vi "DMM_control.vi"(0 "Data in":string, 3 "error in":errorcluster) -> (5 "Data out":string="0.000764", 6 "millisecond timer value":u32, 8 "error out":errorcluster)   [LabVIEW 2011]
doc: "Data in:\n<function><nodes><resolution><range><autozero>\n\nFunction [Integer]\n 0 = DC Volts\n 1 = AC Volts\n 2 = DC Current\n 3 = AC Current\n 4 = Resistance (2 wire)\n 5 = Resistance (4 wire)\n 6 = Frequency\n 7 = Period\n 8 = Diode\n\nNodes [String]\n AB = measueres between a and b\n\nResolution [Integer]\n 0 = 3.5\n 1 = 4.5\n 2 = 5.5\n 3 = 6.5\n\nRange [Float]\n -1 = Autorange\n\nAutoZero [Integer]\n -1 = Auto\n 0 = Off (Default)\n 1 = On\n 2 = Once"
uses:
  <instrlib>/niDMM/nidmm.llb/niDMM Function.ctl
  Server_Globals.vi
  <instrlib>/niDMM/nidmm.llb/niDMM Configure Measurement Digits.vi
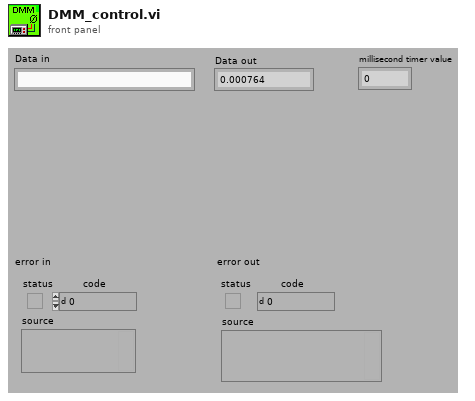
[diagram p1: front panel]
types:
  T1 = cluster{"I/O Settings":u64[], "Instrument Handle":cluster{"5402":refnum<k15>, " 5112":refnum<k15>, "4072":refnum<k15>, "USB":refnum<visa-resource-name>, "4110":refnum<k15>}, "Logfile":refnum<file>, "Log Level":i8, "Clear":i32[], "OS Set":cluster{"instrument handle out":refnum<k15>, "remaining string":string, "Settings":cluster{"Horizontal Conf.":cluster{"Min. Sample rate":dbl, "Reference position":dbl, "Record Length":i16}, "Channel A":cluster{"Enable":bool, "Vertical coupling":dbl, "Vertical range":dbl, "Vertical offset":dbl, "Probe attenuation":dbl}, "Channel B":cluster{"Enable":bool, "Vertical coupling":dbl, "Vertical range":dbl, "Vertical offset":dbl, "Probe attenuation":dbl}, "Trigger":cluster{"Source":enum8{"channel 1", "channel 2", "Imediate", "External trigger"}, "Slope":enum8{"Positive", "Negative"}, "Coupling":enum8{"AC", "DC"}, "Level":dbl, "Holdoff":dbl, "Delay":dbl, " Timeout":dbl, " Mode":enum8{"Normal", "Auto", "Auto Level"}}, "Measurements":cluster{"Measurement 1, Channel":enum8{"Channel 1", "Channel 2", "Channel 3", "Channel 4"}, "Measurement 1, Selection":u16, "Measurement 2, Channel":enum8{"Channel 1", "Channel 2", "Channel 3", "Channel 4"}, "Measurement 2,  Selection":u16, "Measurement 3, Channel":enum8{"Channel 1", "Channel 2", "Channel 3", "Channel 4"}, "Measurement 3, Selection 3":u16}}}, "DC Power Supply":cluster{"0":refnum<k15>, "1":refnum<k15>, "2":refnum<k15>, "3":refnum<k15>, "4":refnum<k15>}, "USB Interface":cluster{"0":refnum<visa-resource-name>, "1":refnum<visa-resource-name>, "2":refnum<visa-resource-name>, "3":refnum<visa-resource-name>, "4":refnum<visa-resource-name>}, "Function Generator":cluster{"0":refnum<k15>, "1":refnum<k15>, "2":refnum<k15>, "3":refnum<k15>, "4":refnum<k15>}, "Digital Multimeter":cluster{"0":refnum<k15>, "1":refnum<k15>, "2":refnum<k15>, "3":refnum<k15>, "4":refnum<k15>}, "Digital Osciliscope":cluster{"0":refnum<k15>, "1":refnum<k15>, "2":refnum<k15>, "3":refnum<k15>, "4":refnum<k15>}, "To M Server":string, "Adres":string[][], "Matrix version":string, "MD5":string, "Digital Multimeter Card 2":cluster{"0":string, "1":string, "2":string, "3":string, "4":string}}
  T2 = cluster{"0":refnum<k15>, "1":refnum<k15>, "2":refnum<k15>, "3":refnum<k15>, "4":refnum<k15>}
  T3 = typedef "niDMM Function.ctl" = enum16{"DC Volts", "AC Volts", "DC Current", "AC Current", "2-wire Resistance", "4-wire Resistance", "Diode", "Frequency", "Period", "AC Volts DC Coupled", "Capacitance", "Inductance", "Temperature"}
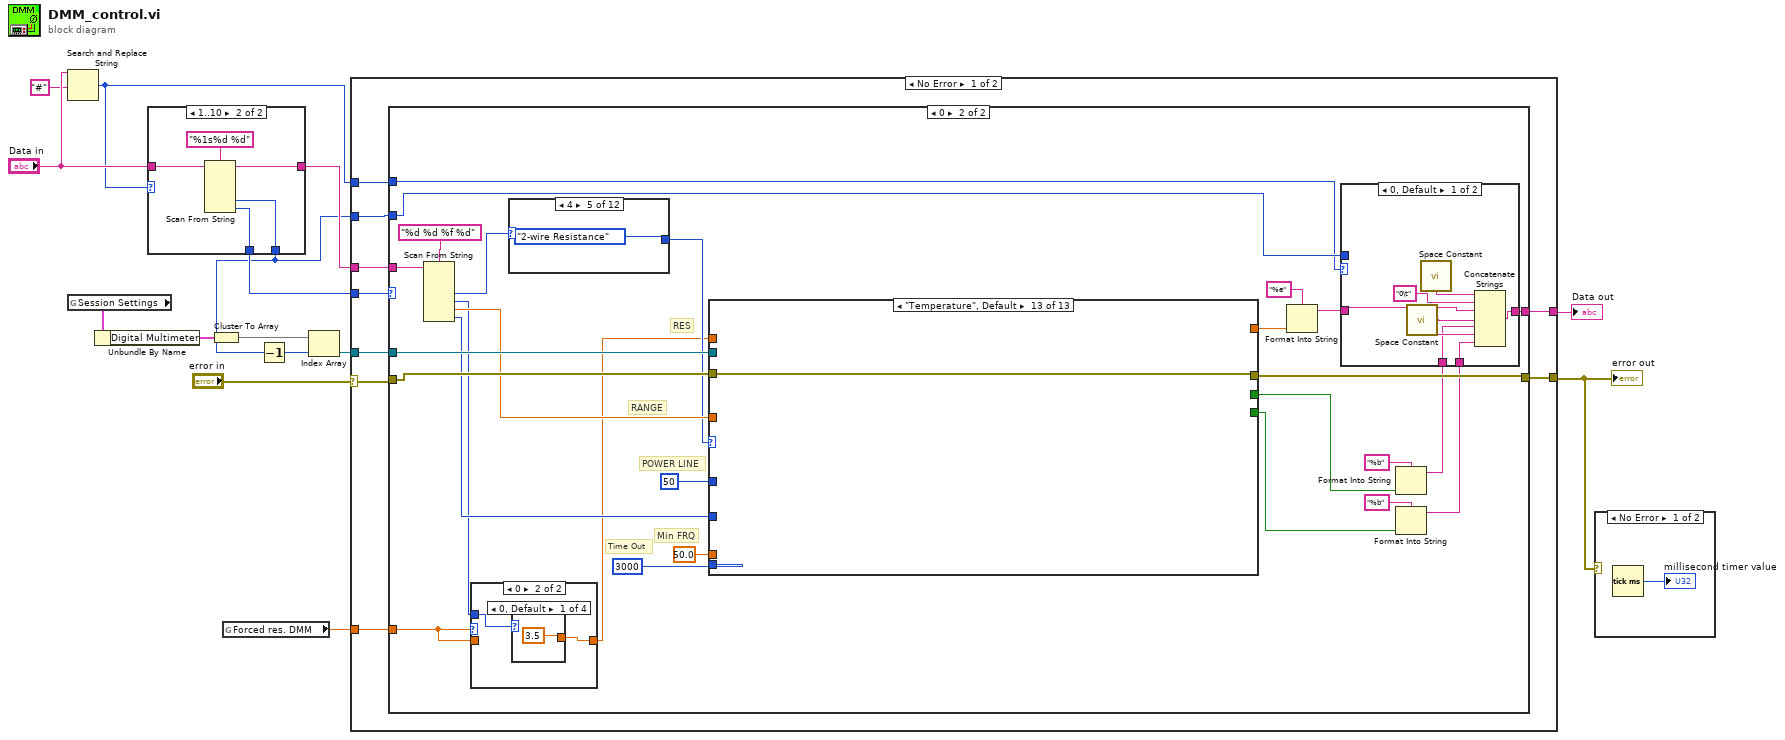
[diagram p0: block diagram]
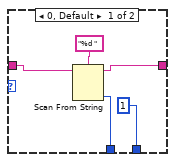
[diagram p2: hidden frame]
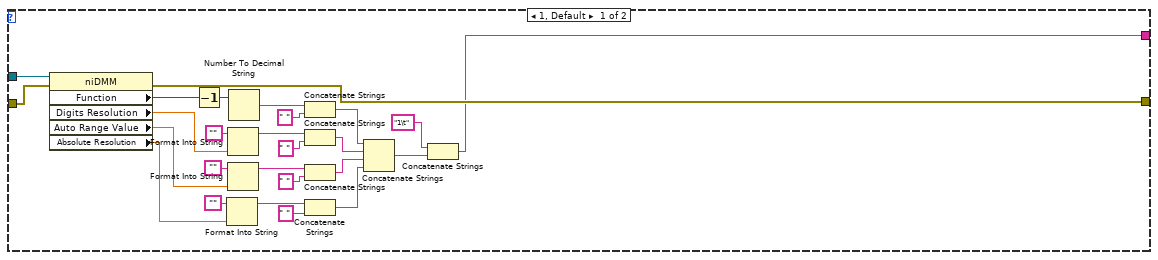
[diagram p4: hidden frame]
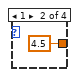
[diagram p6: hidden frame]
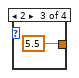
[diagram p7: hidden frame]
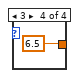
[diagram p8: hidden frame]
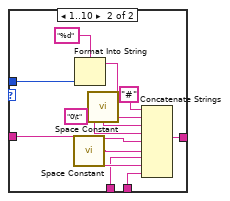
[diagram p9: hidden frame]
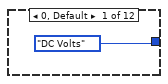
[diagram p10: hidden frame]
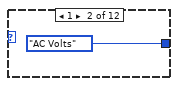
[diagram p11: hidden frame]
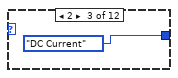
[diagram p12: hidden frame]
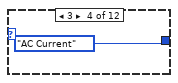
[diagram p13: hidden frame]
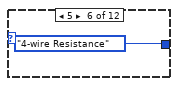
[diagram p14: hidden frame]
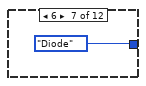
[diagram p15: hidden frame]
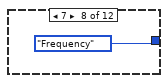
[diagram p16: hidden frame]
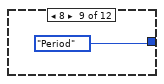
[diagram p17: hidden frame]
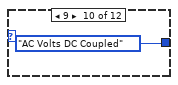
[diagram p18: hidden frame]
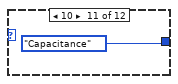
[diagram p19: hidden frame]
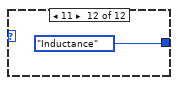
[diagram p20: hidden frame]
diagram:
  w3 = "#"
  n1 = Search and Replace String(input string="Data in", search string=w3, replace string=w3) -> (number of replacements=w2:i32)  [unwired: 5 in, 3 out]
  n2 = global read "Server_Globals.vi" "Session Settings"() -> (w12:T1)
  n3 = Unbundle By Name(w12) -> ("Digital Multimeter"=w11:T2)
  n4 = case shown="1..10" w2 {
    tunnel: [w19 w24] -> w15
    tunnel: [w16 w23] -> w7
    tunnel: [1 w22] -> w5
    tunnel: "Data in" -> [w20 w21]
    frame 0, Default {
      n5 = Scan From String(format string="%d ", input string=w20) -> (remaining string=w19:string, output 1=w16:i32)  [unwired: 3 in, 2 out]
    }
    frame 1..10 {
      n6 = Scan From String(format string="%1s%d %d", input string=w21) -> (remaining string=w24:string, output 2=w22:i32, output 3=w23:i32)  [unwired: 6 in, 2 out]
    }
  }
  n7 = Cluster To Array(cluster=w11) -> (array=w10:refnum<k15>[])
  n8 = global read "DMM_Res" "Forced res. DMM"() -> (w1:dbl)
  n9 = Decrement(x=w5) -> (x-1=w6:i32)
  n10 = Index Array(array=w10, index=w6) -> (element=w9:refnum<k15>)
  n11 = case shown="No Error" "error in" {
    selector: "error in" -> [w29 w360]
    tunnel: [w34 w359] -> w8
    tunnel: w9 -> [w33 _]
    tunnel: w7 -> [w32 _]
    tunnel: w15 -> [w31 _]
    tunnel: [w30 ""] -> w14
    tunnel: w5 -> [w28 _]
    tunnel: w2 -> [w27 _]
    tunnel: w1 -> [w26 _]
    frame No Error {
      n12 = case shown="0" w32 {
        tunnel: [w39 w73] -> w34
        tunnel: w31 -> [_ w84]
        tunnel: w33 -> [w40 w79]
        tunnel: [w35 w86] -> w30
        tunnel: w29 -> [w38 w78]
        tunnel: w28 -> [_ w63]
        tunnel: w27 -> [_ w62]
        tunnel: w26 -> [_ w61]
        frame 1, Default {
          n13 = property class="niDMM"(reference=w40, error in=w38) -> (error out=w39:errorcluster, "Function"=w50:i32, "Digits Resolution"=w48:dbl, "Auto Range Value"=w44:dbl, "Absolute Resolution"=w42:dbl)  [unwired: 1 out]
          n14 = Decrement(x=w50) -> (x-1=w60:i32)
          n15 = Format Into String(initial string="", w42) -> (resulting string=w41:string)  [unwired: 2 in, 1 out]
          n16 = Format Into String(initial string="", w48) -> (resulting string=w45:string)  [unwired: 2 in, 1 out]
          n17 = Format Into String(initial string="", w44) -> (resulting string=w43:string)  [unwired: 2 in, 1 out]
          n18 = Number To Decimal String(number=w60) -> (decimal integer string=w59:string)  [unwired: 1 in]
          n19 = Concatenate Strings(w59, " ") -> (w57:string)
          n20 = Concatenate Strings(w45, " ") -> (w55:string)
          n21 = Concatenate Strings(w43, " ") -> (w53:string)
          n22 = Concatenate Strings(w41, " ") -> (w51:string)
          n23 = Concatenate Strings(w57, w55, w53, w51) -> (w37:string)
          n24 = Concatenate Strings("1\t", w37) -> (w35:string)
        }
        frame 0 {
          # "Time Out"
          # "Min FRQ"
          # "POWER LINE"
          # "RANGE"
          # "RES"
          n25 = Scan From String(format string="%d %d %f %d", input string=w84) -> (output 1=w75:i32, output 2=w65:i32, output 3=w77:dbl, output 4=w76:i32)  [unwired: 6 in, 3 out]
          n26 = case shown="0" w61 {
            tunnel: w65 -> [_ w90]
            tunnel: [w88 w89] -> w64
            tunnel: w61 -> [w88 _]
            frame Default {
            }
            frame 0 {
              n27 = case shown="0, Default" w90 {
                tunnel: [3.5 4.5 5.5 6.5] -> w89
                frame 0, Default {
                }
                frame 1 {
                }
                frame 2 {
                }
                frame 3 {
                }
              }
            }
          }
          n28 = case shown="4" w75 {
            tunnel: [niDMM_Function."DC Volts" ("Measurement Type") niDMM_Function."AC Volts" ("Measurement Type") niDMM_Function."DC Current" ("Measurement Type") niDMM_Function."AC Current" ("Measurement Type") niDMM_Function."2-wire Resistance" ("Measurement Type") niDMM_Function."4-wire Resistance" ("Measurement Type") niDMM_Function."Diode" ("Measurement Type") niDMM_Function."Frequency" ("Measurement Type") niDMM_Function."Period" ("Measurement Type") niDMM_Function."AC Volts DC Coupled" ("Measurement Type") niDMM_Function."Capacitance" ("Measurement Type") niDMM_Function."Inductance" ("Measurement Type")] -> w74
            frame 0, Default {
            }
            frame 1 {
            }
            frame 2 {
            }
            frame 3 {
            }
            frame 4 {
            }
            frame 5 {
            }
            frame 6 {
            }
            frame 7 {
            }
            frame 8 {
            }
            frame 9 {
            }
            frame 10 {
            }
            frame 11 {
            }
          }
          n29 = case shown="\"Temperature\", Default" w74 {
            selector: w74 -> [w142 w166 w191 w213 _ w242 w269 _ _ w298 w317 _ _]
            tunnel: w79 -> [w144 w167 w192 w215 _ w244 w268 _ _ w301 w319 w347 _]
            tunnel: [w139 w161 w194 w219 _ w238 w275 _ _ w294 w324 w354 _] -> w67
            tunnel: [w138 w160 w195 w220 _ w237 w276 _ _ w293 w325 w334 _] -> w70
            tunnel: [w145 w169 w196 w221 w228 w246 w277 w283 w284 w302 w326 w353 w356] -> w73
            tunnel: w78 -> [w141 w164 w177 w214 w228 w243 w270 w283 w284 w300 w320 w346 w356]
            tunnel: 3000 -> [w126 w153 w178 w207 _ w230 w254 _ _ w286 w310 w335 _]
            tunnel: 50 -> [w137 w163 w189 w217 _ w240 w272 _ _ w296 w322 w351 _]
            tunnel: w76 -> [w136 w162 w188 w218 _ w239 w274 _ _ w295 w323 w348 _]
            tunnel: w64 -> [w143 w168 w193 w216 _ w245 w267 _ _ w297 w318 w345 _]
            tunnel: w77 -> [w140 w165 w190 w212 _ w241 w271 _ _ w299 w321 w344 _]
            tunnel: 50.0 -> [w133 _ w185 _ _ _ w263 _ _ _ _ _ _]
            tunnel: [w125 w152 w176 w203 _ w229 w253 _ _ w285 w309 w333 _] -> w72
            frame "AC Volts" {
              n30 = call-poly <instrlib>:"niDMM Config Measurement.vi"("Range"=w140, "Resolution in Digits"=w143, "error in (no error)"=w141, "Function"=w142, "instrument handle"=w144) -> ("error out"=w146:errorcluster, "instrument handle out"=w147:refnum<k15>)  [unwired: 5 in]
              n31 = call <instrlib>:"niDMM Configure Powerline Frequency.vi"("Powerline Frequency"=w137, "error in (no error)"=w146, "instrument handle"=w147) -> ("error out"=w149:errorcluster, "instrument handle out"=w148:refnum<k15>)  [unwired: 7 in]
              n32 = call <instrlib>:"niDMM Configure Auto Zero.vi"("error in (no error)"=w149, "Auto Zero"=w136, "instrument handle"=w148) -> ("error out"=w134:errorcluster, "instrument handle out"=w135:refnum<k15>)  [unwired: 7 in]
              n33 = call <instrlib>:"niDMM Configure AC Bandwidth.vi"("Min Frequency"=w133, "error in (no error)"=w134, "instrument handle"=w135) -> ("error out"=w130:errorcluster, "instrument handle out"=w129:refnum<k15>)  [unwired: 7 in]
              n34 = call <instrlib>:"niDMM Initiate.vi"("error in (no error)"=w130, "instrument handle"=w129) -> ("error out"=w131:errorcluster, "instrument handle out"=w132:refnum<k15>)  [unwired: 8 in]
              n35 = call <instrlib>:"niDMM Fetch.vi"("Maximum Time (msec)"=w126, "error in (no error)"=w131, "instrument handle"=w132) -> ("error out"=w127:errorcluster, "Measurement"=w125:dbl, "instrument handle out"=w128:refnum<k15>)  [unwired: 6 in]
              n36 = call <instrlib>:"niDMM Is Over Range.vi"("error in (no error)"=w127, "Measurement"=w125, "instrument handle"=w128) -> ("error out"=w150:errorcluster, "Over Range?"=w139:bool, "instrument handle out"=w151:refnum<k15>)  [unwired: 6 in]
              n37 = call <instrlib>:"niDMM Is Under Range.vi"("error in (no error)"=w150, "Measurement"=w125, "instrument handle"=w151) -> ("error out"=w145:errorcluster, "Under Range?"=w138:bool)  [unwired: 6 in, 1 out]
            }
            frame "DC Current" {
              n38 = call-poly <instrlib>:"niDMM Config Measurement.vi"("Range"=w165, "Resolution in Digits"=w168, "error in (no error)"=w164, "Function"=w166, "instrument handle"=w167) -> ("error out"=w170:errorcluster, "instrument handle out"=w171:refnum<k15>)  [unwired: 5 in]
              n39 = call <instrlib>:"niDMM Configure Powerline Frequency.vi"("Powerline Frequency"=w163, "error in (no error)"=w170, "instrument handle"=w171) -> ("error out"=w173:errorcluster, "instrument handle out"=w172:refnum<k15>)  [unwired: 7 in]
              n40 = call <instrlib>:"niDMM Configure Auto Zero.vi"("error in (no error)"=w173, "Auto Zero"=w162, "instrument handle"=w172) -> ("error out"=w156:errorcluster, "instrument handle out"=w157:refnum<k15>)  [unwired: 7 in]
              n41 = call <instrlib>:"niDMM Initiate.vi"("error in (no error)"=w156, "instrument handle"=w157) -> ("error out"=w158:errorcluster, "instrument handle out"=w159:refnum<k15>)  [unwired: 8 in]
              n42 = call <instrlib>:"niDMM Fetch.vi"("Maximum Time (msec)"=w153, "error in (no error)"=w158, "instrument handle"=w159) -> ("error out"=w155:errorcluster, "Measurement"=w152:dbl, "instrument handle out"=w154:refnum<k15>)  [unwired: 6 in]
              n43 = call <instrlib>:"niDMM Is Over Range.vi"("error in (no error)"=w155, "Measurement"=w152, "instrument handle"=w154) -> ("error out"=w174:errorcluster, "Over Range?"=w161:bool, "instrument handle out"=w175:refnum<k15>)  [unwired: 6 in]
              n44 = call <instrlib>:"niDMM Is Under Range.vi"("error in (no error)"=w174, "Measurement"=w152, "instrument handle"=w175) -> ("error out"=w169:errorcluster, "Under Range?"=w160:bool)  [unwired: 6 in, 1 out]
            }
            frame "AC Current" {
              n45 = call-poly <instrlib>:"niDMM Config Measurement.vi"("Range"=w190, "Resolution in Digits"=w193, "error in (no error)"=w177, "Function"=w191, "instrument handle"=w192) -> ("error out"=w197:errorcluster, "instrument handle out"=w198:refnum<k15>)  [unwired: 5 in]
              n46 = call <instrlib>:"niDMM Configure Powerline Frequency.vi"("Powerline Frequency"=w189, "error in (no error)"=w197, "instrument handle"=w198) -> ("error out"=w200:errorcluster, "instrument handle out"=w199:refnum<k15>)  [unwired: 7 in]
              n47 = call <instrlib>:"niDMM Configure Auto Zero.vi"("error in (no error)"=w200, "Auto Zero"=w188, "instrument handle"=w199) -> ("error out"=w186:errorcluster, "instrument handle out"=w187:refnum<k15>)  [unwired: 7 in]
              n48 = call <instrlib>:"niDMM Configure AC Bandwidth.vi"("Min Frequency"=w185, "error in (no error)"=w186, "instrument handle"=w187) -> ("error out"=w181:errorcluster, "instrument handle out"=w182:refnum<k15>)  [unwired: 7 in]
              n49 = call <instrlib>:"niDMM Initiate.vi"("error in (no error)"=w181, "instrument handle"=w182) -> ("error out"=w183:errorcluster, "instrument handle out"=w184:refnum<k15>)  [unwired: 8 in]
              n50 = call <instrlib>:"niDMM Fetch.vi"("Maximum Time (msec)"=w178, "error in (no error)"=w183, "instrument handle"=w184) -> ("error out"=w180:errorcluster, "Measurement"=w176:dbl, "instrument handle out"=w179:refnum<k15>)  [unwired: 6 in]
              n51 = call <instrlib>:"niDMM Is Over Range.vi"("error in (no error)"=w180, "Measurement"=w176, "instrument handle"=w179) -> ("error out"=w201:errorcluster, "Over Range?"=w194:bool, "instrument handle out"=w202:refnum<k15>)  [unwired: 6 in]
              n52 = call <instrlib>:"niDMM Is Under Range.vi"("error in (no error)"=w201, "Measurement"=w176, "instrument handle"=w202) -> ("error out"=w196:errorcluster, "Under Range?"=w195:bool)  [unwired: 6 in, 1 out]
            }
            frame "2-wire Resistance" {
              n53 = call-poly <instrlib>:"niDMM Config Measurement.vi"("Range"=w212, "Resolution in Digits"=w216, "error in (no error)"=w214, "Function"=w213, "instrument handle"=w215) -> ("error out"=w222:errorcluster, "instrument handle out"=w223:refnum<k15>)  [unwired: 5 in]
              n54 = call <instrlib>:"niDMM Configure Powerline Frequency.vi"("Powerline Frequency"=w217, "error in (no error)"=w222, "instrument handle"=w223) -> ("error out"=w225:errorcluster, "instrument handle out"=w224:refnum<k15>)  [unwired: 7 in]
              n55 = call <instrlib>:"niDMM Configure Auto Zero.vi"("error in (no error)"=w225, "Auto Zero"=w218, "instrument handle"=w224) -> ("error out"=w205:errorcluster, "instrument handle out"=w206:refnum<k15>)  [unwired: 7 in]
              n56 = call <instrlib>:"niDMM Initiate.vi"("error in (no error)"=w205, "instrument handle"=w206) -> ("error out"=w210:errorcluster, "instrument handle out"=w211:refnum<k15>)  [unwired: 8 in]
              n57 = call <instrlib>:"niDMM Fetch.vi"("Maximum Time (msec)"=w207, "error in (no error)"=w210, "instrument handle"=w211) -> ("error out"=w208:errorcluster, "Measurement"=w204:dbl, "instrument handle out"=w209:refnum<k15>)  [unwired: 6 in]
              n58 = call <instrlib>:"niDMM Is Over Range.vi"("error in (no error)"=w208, "Measurement"=w204, "instrument handle"=w209) -> ("error out"=w226:errorcluster, "Over Range?"=w219:bool, "instrument handle out"=w227:refnum<k15>)  [unwired: 6 in]
              n59 = call <instrlib>:"niDMM Is Under Range.vi"("error in (no error)"=w226, "Measurement"=w204, "instrument handle"=w227) -> ("error out"=w221:errorcluster, "Under Range?"=w220:bool)  [unwired: 6 in, 1 out]
              n60 = Absolute Value(x=w204) -> (abs(x)=w203:dbl)
            }
            frame "4-wire Resistance" {
              # "This is not suported by the matrix."
            }
            frame "Diode" {
              n61 = call-poly <instrlib>:"niDMM Config Measurement.vi"("Range"=w241, "Resolution in Digits"=w245, "error in (no error)"=w243, "Function"=w242, "instrument handle"=w244) -> ("error out"=w247:errorcluster, "instrument handle out"=w248:refnum<k15>)  [unwired: 5 in]
              n62 = call <instrlib>:"niDMM Configure Powerline Frequency.vi"("Powerline Frequency"=w240, "error in (no error)"=w247, "instrument handle"=w248) -> ("error out"=w250:errorcluster, "instrument handle out"=w249:refnum<k15>)  [unwired: 7 in]
              n63 = call <instrlib>:"niDMM Configure Auto Zero.vi"("error in (no error)"=w250, "Auto Zero"=w239, "instrument handle"=w249) -> ("error out"=w233:errorcluster, "instrument handle out"=w234:refnum<k15>)  [unwired: 7 in]
              n64 = call <instrlib>:"niDMM Initiate.vi"("error in (no error)"=w233, "instrument handle"=w234) -> ("error out"=w235:errorcluster, "instrument handle out"=w236:refnum<k15>)  [unwired: 8 in]
              n65 = call <instrlib>:"niDMM Fetch.vi"("Maximum Time (msec)"=w230, "error in (no error)"=w235, "instrument handle"=w236) -> ("error out"=w231:errorcluster, "Measurement"=w229:dbl, "instrument handle out"=w232:refnum<k15>)  [unwired: 6 in]
              n66 = call <instrlib>:"niDMM Is Over Range.vi"("error in (no error)"=w231, "Measurement"=w229, "instrument handle"=w232) -> ("error out"=w251:errorcluster, "Over Range?"=w238:bool, "instrument handle out"=w252:refnum<k15>)  [unwired: 6 in]
              n67 = call <instrlib>:"niDMM Is Under Range.vi"("error in (no error)"=w251, "Measurement"=w229, "instrument handle"=w252) -> ("error out"=w246:errorcluster, "Under Range?"=w237:bool)  [unwired: 6 in, 1 out]
            }
            frame "Frequency" {
              w266 = 0.04
              w264 = 0
              n68 = call-poly <instrlib>:"niDMM Config Measurement.vi"("Range"=w271, "Resolution in Digits"=w267, "error in (no error)"=w270, "Function"=w269, "instrument handle"=w268) -> ("error out"=w278:errorcluster, "instrument handle out"=w279:refnum<k15>)  [unwired: 5 in]
              n69 = call <instrlib>:"niDMM Configure Powerline Frequency.vi"("Powerline Frequency"=w272, "error in (no error)"=w278, "instrument handle"=w279) -> ("error out"=w280:errorcluster, "instrument handle out"=w273:refnum<k15>)  [unwired: 7 in]
              n70 = call <instrlib>:"niDMM Configure Auto Zero.vi"("error in (no error)"=w280, "Auto Zero"=w274, "instrument handle"=w273) -> ("error out"=w261:errorcluster, "instrument handle out"=w262:refnum<k15>)  [unwired: 7 in]
              n71 = property class="niDMM"(reference=w262, error in=w261, "Settle Time"=w266, "Aperture Time"=w266, "Number Of Averages"=1, "Trigger Delay"=w264, "ADC Calibration"=w264, "Min Frequency"=w263) -> (reference out=w260:refnum<k15>, error out=w259:errorcluster)
              n72 = call <instrlib>:"niDMM Initiate.vi"("error in (no error)"=w259, "instrument handle"=w260) -> ("error out"=w255:errorcluster, "instrument handle out"=w256:refnum<k15>)  [unwired: 8 in]
              n73 = call <instrlib>:"niDMM Fetch.vi"("Maximum Time (msec)"=w254, "error in (no error)"=w255, "instrument handle"=w256) -> ("error out"=w258:errorcluster, "Measurement"=w253:dbl, "instrument handle out"=w257:refnum<k15>)  [unwired: 6 in]
              n74 = call <instrlib>:"niDMM Is Over Range.vi"("error in (no error)"=w258, "Measurement"=w253, "instrument handle"=w257) -> ("error out"=w281:errorcluster, "Over Range?"=w275:bool, "instrument handle out"=w282:refnum<k15>)  [unwired: 6 in]
              n75 = call <instrlib>:"niDMM Is Under Range.vi"("error in (no error)"=w281, "Measurement"=w253, "instrument handle"=w282) -> ("error out"=w277:errorcluster, "Under Range?"=w276:bool)  [unwired: 6 in, 1 out]
            }
            frame "Period" {
            }
            frame "AC Volts DC Coupled" {
            }
            frame "Capacitance" {
              n76 = call-poly <instrlib>:"niDMM Config Measurement.vi"("Range"=w299, "Resolution in Digits"=w297, "error in (no error)"=w300, "Function"=w298, "instrument handle"=w301) -> ("error out"=w303:errorcluster, "instrument handle out"=w304:refnum<k15>)  [unwired: 5 in]
              n77 = call <instrlib>:"niDMM Configure Powerline Frequency.vi"("Powerline Frequency"=w296, "error in (no error)"=w303, "instrument handle"=w304) -> ("error out"=w306:errorcluster, "instrument handle out"=w305:refnum<k15>)  [unwired: 7 in]
              n78 = call <instrlib>:"niDMM Configure Auto Zero.vi"("error in (no error)"=w306, "Auto Zero"=w295, "instrument handle"=w305) -> ("error out"=w289:errorcluster, "instrument handle out"=w290:refnum<k15>)  [unwired: 7 in]
              n79 = call <instrlib>:"niDMM Initiate.vi"("error in (no error)"=w289, "instrument handle"=w290) -> ("error out"=w291:errorcluster, "instrument handle out"=w292:refnum<k15>)  [unwired: 8 in]
              n80 = call <instrlib>:"niDMM Fetch.vi"("Maximum Time (msec)"=w286, "error in (no error)"=w291, "instrument handle"=w292) -> ("error out"=w288:errorcluster, "Measurement"=w285:dbl, "instrument handle out"=w287:refnum<k15>)  [unwired: 6 in]
              n81 = call <instrlib>:"niDMM Is Over Range.vi"("error in (no error)"=w288, "Measurement"=w285, "instrument handle"=w287) -> ("error out"=w307:errorcluster, "Over Range?"=w294:bool, "instrument handle out"=w308:refnum<k15>)  [unwired: 6 in]
              n82 = call <instrlib>:"niDMM Is Under Range.vi"("error in (no error)"=w307, "Measurement"=w285, "instrument handle"=w308) -> ("error out"=w302:errorcluster, "Under Range?"=w293:bool)  [unwired: 6 in, 1 out]
            }
            frame "Inductance" {
              n83 = call-poly <instrlib>:"niDMM Config Measurement.vi"("Range"=w321, "Resolution in Digits"=w318, "error in (no error)"=w320, "Function"=w317, "instrument handle"=w319) -> ("error out"=w327:errorcluster, "instrument handle out"=w328:refnum<k15>)  [unwired: 5 in]
              n84 = call <instrlib>:"niDMM Configure Powerline Frequency.vi"("Powerline Frequency"=w322, "error in (no error)"=w327, "instrument handle"=w328) -> ("error out"=w330:errorcluster, "instrument handle out"=w329:refnum<k15>)  [unwired: 7 in]
              n85 = call <instrlib>:"niDMM Configure Auto Zero.vi"("error in (no error)"=w330, "Auto Zero"=w323, "instrument handle"=w329) -> ("error out"=w311:errorcluster, "instrument handle out"=w312:refnum<k15>)  [unwired: 7 in]
              n86 = call <instrlib>:"niDMM Initiate.vi"("error in (no error)"=w311, "instrument handle"=w312) -> ("error out"=w315:errorcluster, "instrument handle out"=w316:refnum<k15>)  [unwired: 8 in]
              n87 = call <instrlib>:"niDMM Fetch.vi"("Maximum Time (msec)"=w310, "error in (no error)"=w315, "instrument handle"=w316) -> ("error out"=w313:errorcluster, "Measurement"=w309:dbl, "instrument handle out"=w314:refnum<k15>)  [unwired: 6 in]
              n88 = call <instrlib>:"niDMM Is Over Range.vi"("error in (no error)"=w313, "Measurement"=w309, "instrument handle"=w314) -> ("error out"=w331:errorcluster, "Over Range?"=w324:bool, "instrument handle out"=w332:refnum<k15>)  [unwired: 6 in]
              n89 = call <instrlib>:"niDMM Is Under Range.vi"("error in (no error)"=w331, "Measurement"=w309, "instrument handle"=w332) -> ("error out"=w326:errorcluster, "Under Range?"=w325:bool)  [unwired: 6 in, 1 out]
            }
            frame "DC Volts" {
              n90 = call-poly <instrlib>:"niDMM Config Measurement.vi"("Range"=w344, "Resolution in Digits"=w345, "error in (no error)"=w346, "instrument handle"=w347) -> ("error out"=w342:errorcluster, "instrument handle out"=w343:refnum<k15>)  [unwired: 6 in]
              n91 = call <instrlib>:"niDMM Configure Powerline Frequency.vi"("Powerline Frequency"=w351, "error in (no error)"=w342, "instrument handle"=w343) -> ("error out"=w350:errorcluster, "instrument handle out"=w349:refnum<k15>)  [unwired: 7 in]
              n92 = call <instrlib>:"niDMM Configure Auto Zero.vi"("error in (no error)"=w350, "Auto Zero"=w348, "instrument handle"=w349) -> ("error out"=w338:errorcluster, "instrument handle out"=w339:refnum<k15>)  [unwired: 7 in]
              n93 = call <instrlib>:"niDMM Initiate.vi"("error in (no error)"=w338, "instrument handle"=w339) -> ("error out"=w340:errorcluster, "instrument handle out"=w341:refnum<k15>)  [unwired: 8 in]
              n94 = call <instrlib>:"niDMM Fetch.vi"("Maximum Time (msec)"=w335, "error in (no error)"=w340, "instrument handle"=w341) -> ("error out"=w337:errorcluster, "Measurement"=w333:dbl, "instrument handle out"=w336:refnum<k15>)  [unwired: 6 in]
              n95 = call <instrlib>:"niDMM Is Over Range.vi"("error in (no error)"=w337, "Measurement"=w333, "instrument handle"=w336) -> ("error out"=w352:errorcluster, "Over Range?"=w354:bool, "instrument handle out"=w355:refnum<k15>)  [unwired: 6 in]
              n96 = call <instrlib>:"niDMM Is Under Range.vi"("error in (no error)"=w352, "Measurement"=w333, "instrument handle"=w355) -> ("error out"=w353:errorcluster, "Under Range?"=w334:bool)  [unwired: 6 in, 1 out]
            }
            frame "Temperature", Default {
            }
          }
          n97 = Format Into String(format string="%e", w72) -> (resulting string=w87:string)  [unwired: 2 in, 1 out]
          n98 = Format Into String(format string="%b", w70) -> (resulting string=w69:string)  [unwired: 2 in, 1 out]
          n99 = Format Into String(format string="%b", w67) -> (resulting string=w66:string)  [unwired: 2 in, 1 out]
          n100 = case shown="0, Default" w62 {
            tunnel: w87 -> [w96 w111]
            tunnel: [w95 w110] -> w86
            tunnel: w69 -> [w97 w108]
            tunnel: w66 -> [w98 w107]
            tunnel: w63 -> [_ w105]
            frame 0, Default {
              n101 = call <vilib>:"Space Constant.vi"() -> ("String"=w100:string)
              n102 = call <vilib>:"Space Constant.vi"() -> ("String"=w101:string)
              n103 = Concatenate Strings(w101, "0\t", w96, w100, w97, w100, w98) -> (w95:string)
            }
            frame 1..10 {
              n104 = call <vilib>:"Space Constant.vi"() -> ("String"=w109:string)
              n105 = Format Into String(format string="%d", w105) -> (resulting string=w103:string)  [unwired: 2 in, 1 out]
              n106 = call <vilib>:"Space Constant.vi"() -> ("String"=w102:string)
              n107 = Concatenate Strings("#", w103, w102, "0\t", w111, w109, w108, w109, w107) -> (w110:string)
            }
          }
        }
      }
    }
    frame Error {
      n108 = call "Error Converter.vi"("error in (no error)"=w360, "String to add to error message"="Message from 4072 DMM:" ("String to add message")) -> ("error out (no error)"=w359:errorcluster)
    }
  }
  "error out" <- w8
  "Data out" <- w14
  n109 = case shown="No Error" w8 {
    frame No Error {
      n110 = Tick Count (ms)() -> (millisecond timer value=→"millisecond timer value":u32)
    }
    frame Error {
    }
  }
